vi "deleteFileCategory.vi"(1 "VarableID":T1) -> ()   [LabVIEW 2010]
uses:
  VarableID.ctl
  GlobalCostants.vi
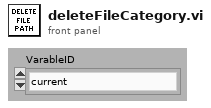
[diagram p1: front panel]
types:
  T1 = typedef "VarableID.ctl" = enum16{"current", "voltage", "power", "PF"}
  T2 = typedef "VarableStruct.ctl" = cluster{"Name":string, "StorageRefnum":refnum<file>, "Command":string, "IsDetecting":bool, "VarableID":T1}
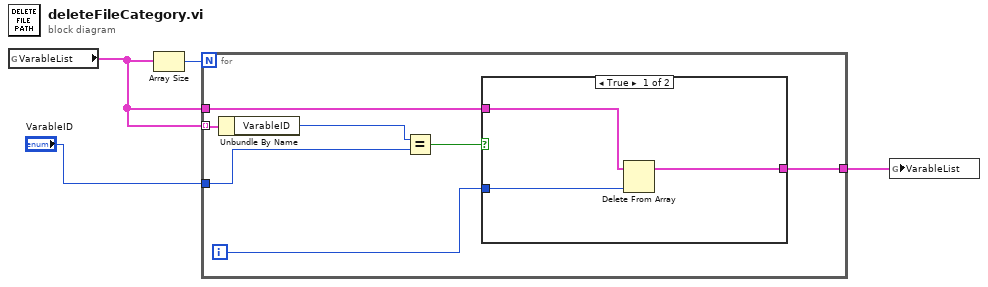
[diagram p0: block diagram]
diagram:
  n1 = global read "GlobalCostants.vi" "VarableList"() -> (w3:T2[])
  n2 = Array Size(array=w3) -> (size(s)=w4:i32)
  n3 = for {
    N: w4 -> [_]
    tunnel: "VarableID" -> [w6]
    tunnel: w3 -> [w7] mode=indexing
    tunnel: w3 -> [w10]
    tunnel: [w8] -> w1
    i -> [w9]
    n4 = Unbundle By Name(w7) -> ("VarableID"=w5:T1)
    n5 = Equal?(x=w5, y=w6) -> (x = y?=w11:bool)
    n6 = case shown="True" w11 {
      tunnel: w10 -> [w14 w15]
      tunnel: w9 -> [w13 _]
      tunnel: [w12 w15] -> w8
      frame True {
        n7 = Delete From Array(array=w14, index=w13) -> (array with subset deleted=w12:T2[])  [unwired: 1 in, 1 out]
      }
      frame False {
      }
    }
  }
  n8 = global write "GlobalCostants.vi" "VarableList"(w1) -> ()
